vi "Delete Object.vi"(8 "error in (no error)":errorcluster, 9 "Version ID":string, 10 "Object Key":string, 11 "Bucket in":refnum<class "Bucket.lvclass">) -> (0 "error out":errorcluster, 3 "Bucket out":refnum<class "Bucket.lvclass">)   [LabVIEW 2015, in "NI_AWS_S3.lvlib" / "Bucket.lvclass"]
doc: "The DELETE operation removes the null version (if there is one) of an object and inserts a delete marker, which becomes the current version of the object."
uses:
  Bucket.lvclass
  Core/HTTP Request/Request Options.ctl
  Core/HTTP Request/Name Value Pair.ctl
  Core/HTTP Request/Region handling.ctl
  Core/HTTP Request/URL formatting.ctl
  Bucket.lvclass/Bucket.ctl
  Read Name.vi
  Core/HTTP Request/HTTP Request.lvclass
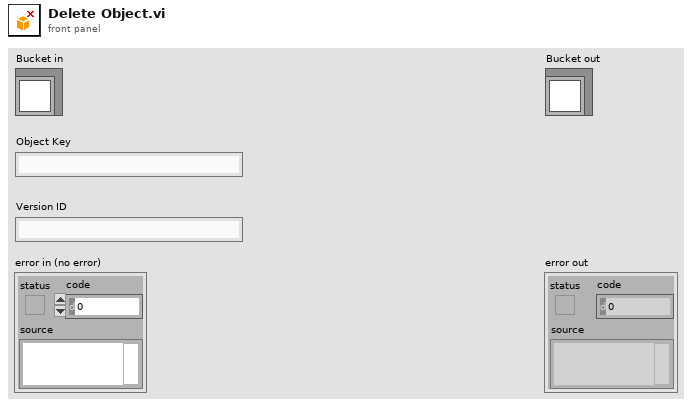
[diagram p1: front panel]
types:
  T1 = typedef "NI_AWS_Core.lvlib/HTTP Request.lvclass/Region handling.ctl" = enum16{"use region everywhere", "use region (authentication only)", "use region (URL only)", "ignore region everwhere"}
  T2 = typedef "NI_AWS_Core.lvlib/HTTP Request.lvclass/Request Options.ctl" = cluster{"request headers":T3[], "request parameters":T3[], "request body":string, "region handling":T1, "URL formatting":T4}
  T3 = typedef "NI_AWS_Core.lvlib/HTTP Request.lvclass/Name Value Pair.ctl" = cluster{"name":string, "value":string}
  T4 = typedef "NI_AWS_Core.lvlib/HTTP Request.lvclass/URL formatting.ctl" = enum16{"region-", "region."}
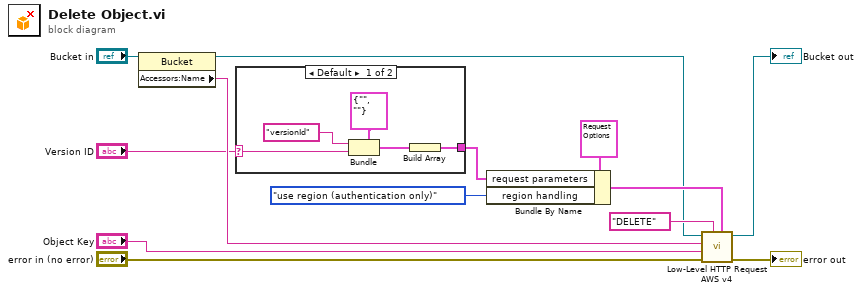
[diagram p0: block diagram]
diagram:
  n1 = property class="Bucket"(reference="Bucket in") -> (reference out=w3:refnum<class "Bucket.lvclass">, "Accessors:Name"=w12:string)  [unwired: 1 in, 1 out]
  n2 = case shown="Default" "Version ID" {
    selector: "Version ID" -> [w15 _]
    tunnel: [w16 _] -> w1
    frame Default {
      n3 = Bundle(cluster=T3 {"name"="", "value"=""} ("Name Value Pair"), "name"="versionId", "value"=w15) -> (w17:T3)
      n4 = Build Array(w17) -> (w16:T3[])
    }
    frame "" {
    }
  }
  n5 = Bundle By Name(cluster=T2 {"request headers"=[], "request parameters"=[], "request body"="", "region handling"=enum."use region everywhere", "URL formatting"=enum."region."} ("Request Options"), "request parameters"=w1, "region handling"=Region_handling."use region (authentication only)") -> (w4:T2)
  n6 = call "Low-Level HTTP Request AWS v4.vi"("Request Options"=w4, "HTTP-Verb"="DELETE", "error in (no error)"="error in (no error)", "URL Suffix"="Object Key", "URL Prefix"=w12, "AWS Core in"=w3) -> ("error out"=→"error out":errorcluster, "AWS Core out"=→"Bucket out":refnum<class "Bucket.lvclass">)  [unwired: 2 in, 2 out]
